vi "Set Node Status Changed.vi"(8 "error in":errorcluster, 10 "Node Status Changed":refnum<user-event>, 11 "Node Guard in":refnum<class "Node Guard.lvclass">) -> (0 "error out":errorcluster, 3 "Node Guard out":refnum<class "Node Guard.lvclass">)   [LabVIEW 2020, in "CANopen.lvlib" / "Network Management.lvlib" / "Node Guard.lvlib" / "Node Guard.lvclass"]
uses:
  Node Guard.lvclass
  Node Guard.lvclass/Node Guard.ctl
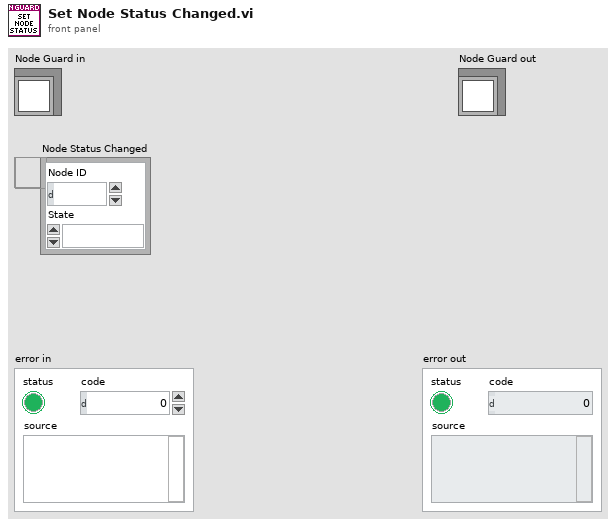
[diagram p1: front panel]
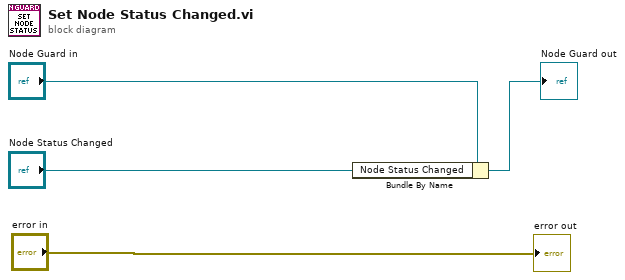
[diagram p0: block diagram]
diagram:
  n1 = Bundle By Name(cluster="Node Guard in", "Node Status Changed"="Node Status Changed") -> (→"Node Guard out":refnum<class "Node Guard.lvclass">)
  "error out" <- "error in"
